vi "GT_LmtSns.vi"(1 "Sense":u16, 2 "rtn_In":cluster{"rtn":i16, "Func":string}) -> (0 "rtn_Out":cluster{"rtn":i16, "Func":string})   [LabVIEW 2014]
uses:
  VC6/gts.dll
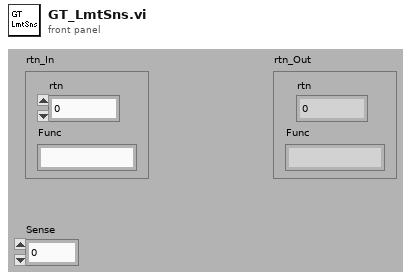
[diagram p1: front panel]
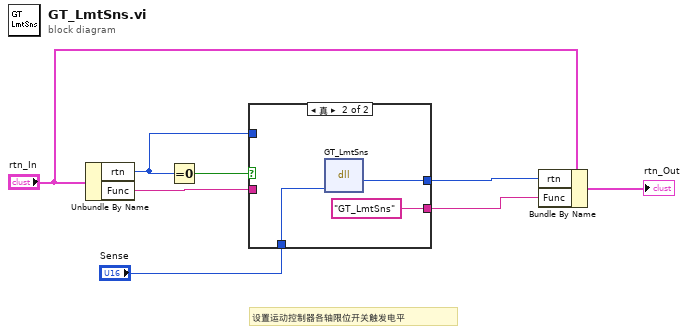
[diagram p0: block diagram]
diagram:
  # "设置运动控制器各轴限位开关触发电平"
  n1 = Unbundle By Name("rtn_In") -> ("rtn"=w2:i16, "Func"=w6:string)
  n2 = Equal To 0?(x=w2) -> (x = 0?=w8:bool)
  n3 = case shown="真" w8 {
    tunnel: "Sense" -> [_ w13]
    tunnel: w6 -> [w9 _]
    tunnel: [w10 w12] -> w4
    tunnel: [w9 "GT_LmtSns" ("Func")] -> w3
    tunnel: w2 -> [w10 _]
    frame False {
    }
    frame True {
      n4 = dll-call lib="PTH2Iabs E+Win7系统AC-800标准版源程序-20170822gts85VC6gts.dll" fn="GT_LmtSns"("Sense"=w13) -> ("rtn"=w12:i16)  [unwired: 4 in, 2 out]
    }
  }
  n5 = Bundle By Name(cluster="rtn_In", "rtn"=w4, "Func"=w3) -> (→"rtn_Out":cluster{"rtn":i16, "Func":string})
